vi "All IOs.vi"() -> ()   [LabVIEW 2015]
uses:
  <vilib>/rvi/Emulation/niFpgaGetClockAttributes.vi
  <vilib>/rvi/Emulation/niFpgaSctlEmulationGetInTimedLoop.vi
  <vilib>/rvi/Emulation/niFpgaEmulationReportErrorSimple.vi
  <vilib>/rvi/eio/common/nirviEmuTemplateMethod_errors.vi
  <vilib>/rvi/Emulation/niFpgaCriticalErrorInLSC.vi
  <vilib>/rvi/Emulation/niFpgaProcessEmulError.vi
  <vilib>/eio/EIONode/EIONode.xnode
panel:
  out "Time of flight":T1
  in  "6DOF robot arm controls":T2={"Axis  1 (base)"=1250, "Axis 2"=1600, "Axis 3"=1000, "Axis 4"=1900, "Axis 5"=1300, "Axis 6 (claw)"=1800} {"Axis 6 (claw)" min=500 max=2000; "Axis 5" min=500 max=2000; "Axis 4" min=500 max=2000; "Axis 3" min=500 max=2000; "Axis 2" min=500 max=2000; "Axis  1 (base)" min=500 max=2000}
  out "Lipo Battery Voltage":i16
  out "PIR 2":bool
  in  "FL":bool
  in  "BL":bool
  in  "FR":bool
  in  "BR":bool
  in  "On-board LED Brightness":T3 {"LED3 Brightness" max=100; "LED2 Brightness" max=100; "LED1 Brightness" max=100; "LED0 Brightness" max=100}
  out "Accelerometer":T4
  out "Button0":bool
  out "PIR":bool
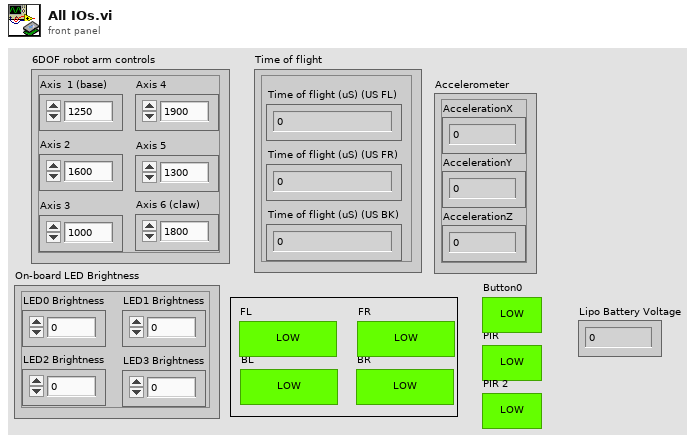
[diagram p1: front panel]
types:
  T1 = cluster{"Time of flight (uS) (US FL)":u32, "Time of flight (uS) (US FR)":u32, "Time of flight (uS) (US BK)":u32}
  T2 = cluster{"Axis  1 (base)":i16, "Axis 2":i16, "Axis 3":i16, "Axis 4":i16, "Axis 5":i16, "Axis 6 (claw)":i16}
  T3 = cluster{"LED0 Brightness":u8, "LED1 Brightness":u8, "LED2 Brightness":u8, "LED3 Brightness":u8}
  T4 = cluster{"AccelerationX":i16, "AccelerationY":i16, "AccelerationZ":i16}
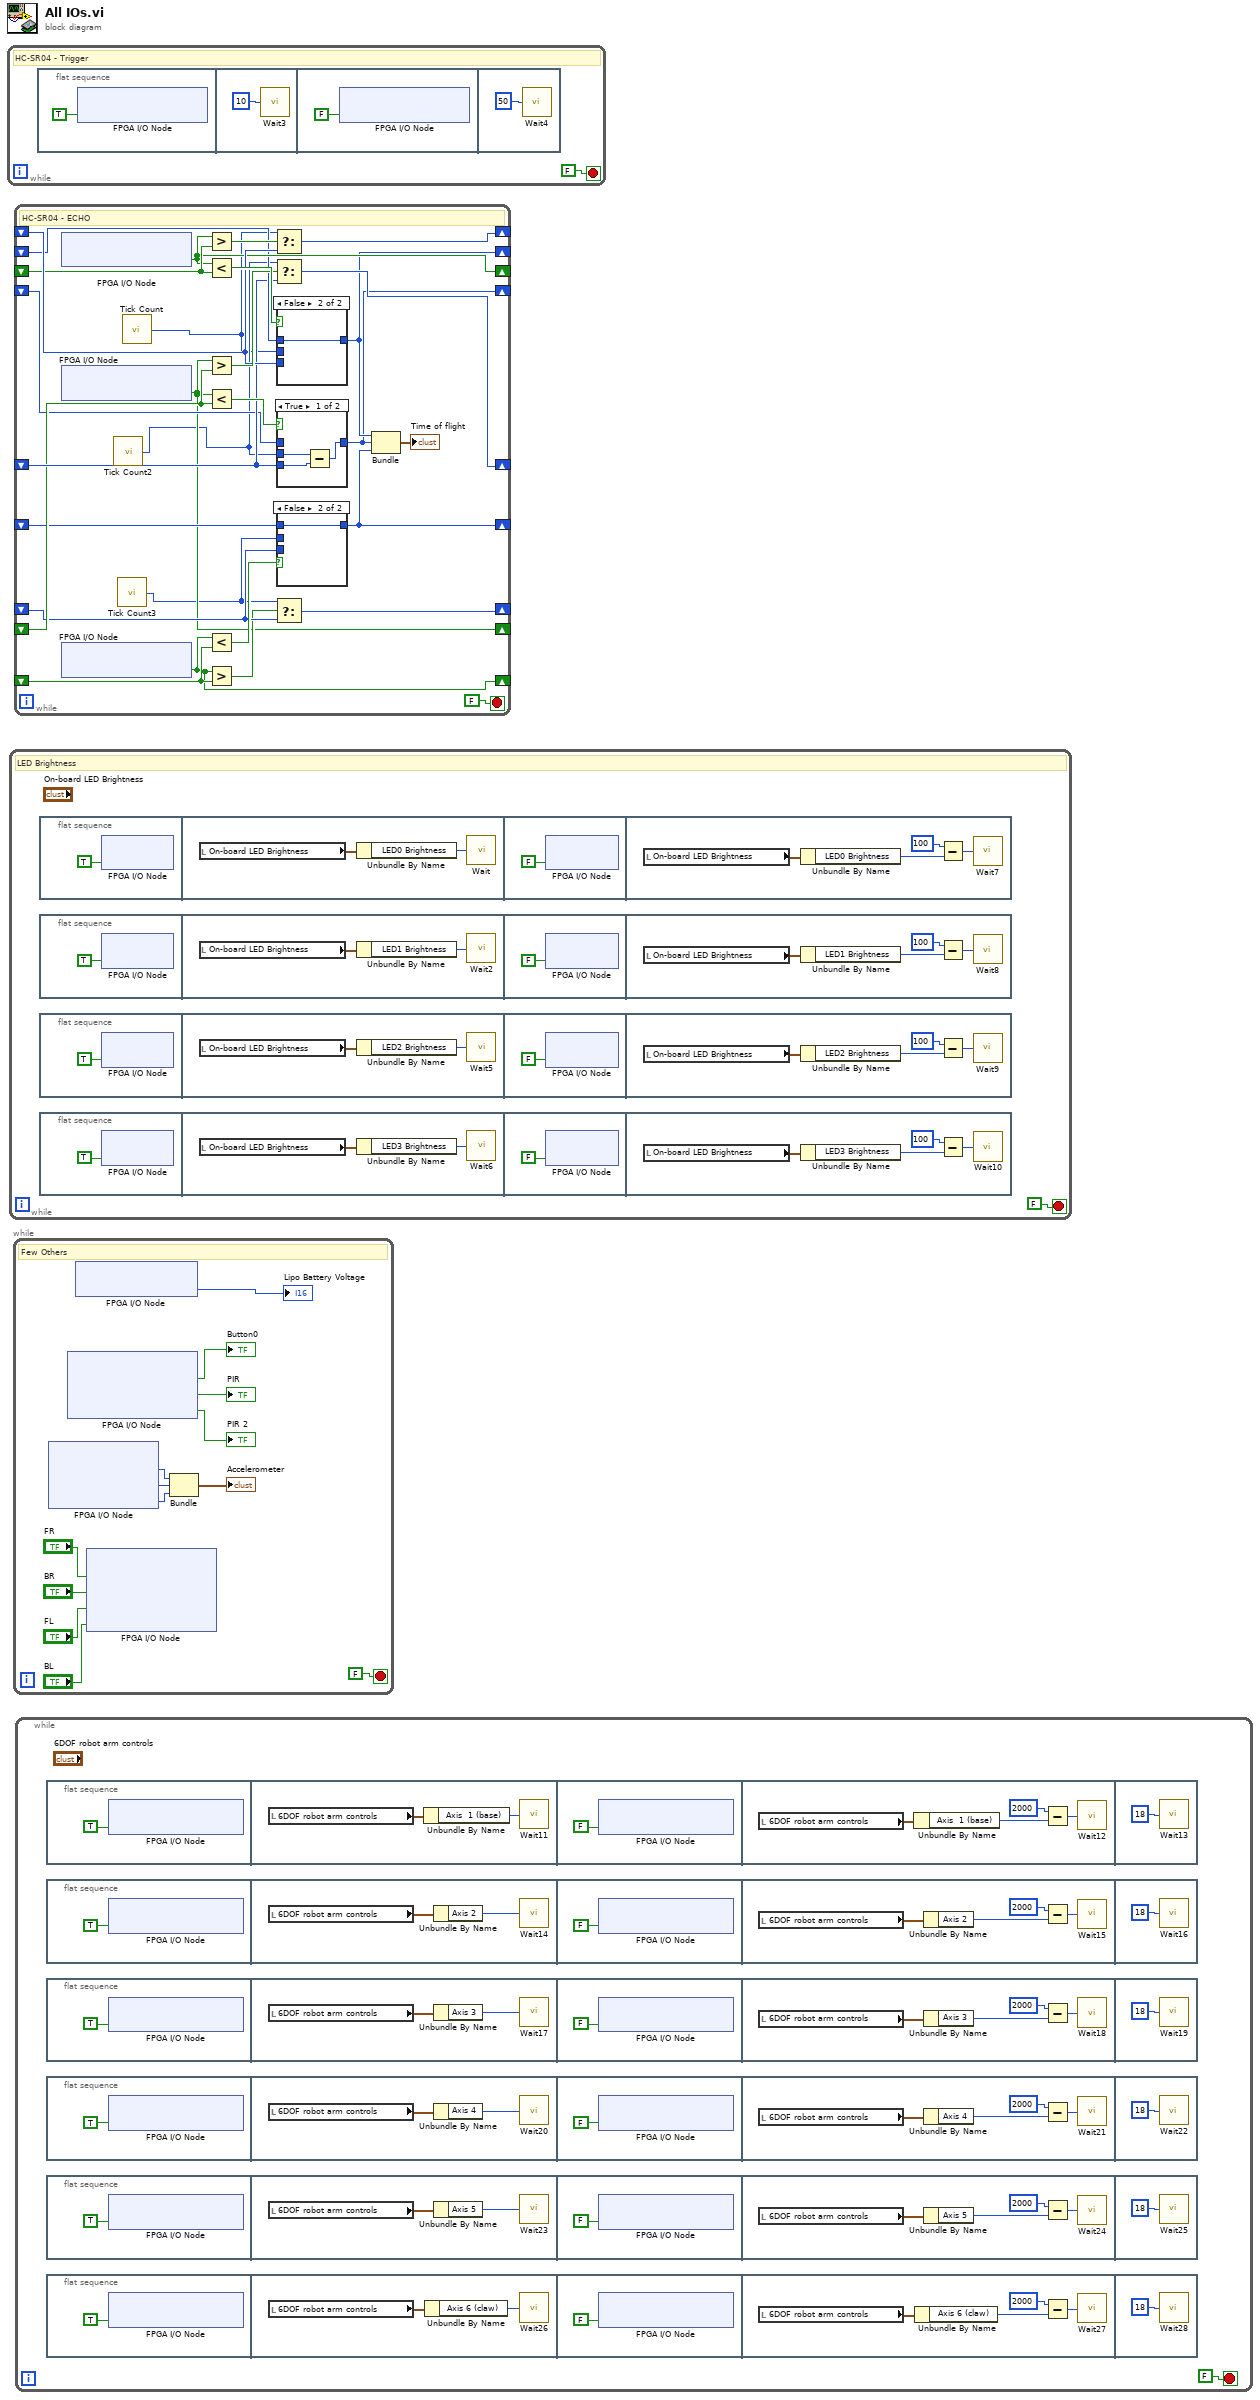
[diagram p0: block diagram]
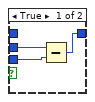
[diagram p2: hidden frame]
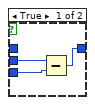
[diagram p3: hidden frame]
diagram:
  n1 = while {
    stop <- FALSE stop-if-true
    # "HC-SR04 - Trigger"
    n2 = flat-sequence {
      frame #0 {
        n3 = xnode "FPGA I/O Node"("ConnectorC/DIO0"=TRUE ("ConnectorC/DIO6")) -> ()  [unwired: 1 in, 1 out]
      }
      frame #1 {
        n4 = call "Wait3"("Count(uSec)"=u32 10) -> ()  [unwired: 1 out]
      }
      frame #2 {
        n5 = xnode "FPGA I/O Node"("ConnectorC/DIO0"=FALSE ("ConnectorC/DIO6")) -> ()  [unwired: 1 in, 1 out]
      }
      frame #3 {
        n6 = call "Wait4"("Count(mSec)"=i16 50) -> ()  [unwired: 1 out]
      }
    }
  }
  n7 = while {
    stop <- FALSE stop-if-true
    # "LED Brightness"
    n8 = flat-sequence {
      frame #0 {
        n9 = xnode "FPGA I/O Node"("LED0"=TRUE) -> ()  [unwired: 1 in, 1 out]
      }
      frame #1 {
        n10 = local read "On-board LED Brightness"() -> (w33:T3)
        n11 = Unbundle By Name(w33) -> ("LED0 Brightness"=w32:u8)
        n12 = call "Wait"("Count(uSec)"=w32) -> ()  [unwired: 1 out]
      }
      frame #2 {
        n13 = xnode "FPGA I/O Node"("LED0"=FALSE) -> ()  [unwired: 1 in, 1 out]
      }
      frame #3 {
        n14 = local read "On-board LED Brightness"() -> (w38:T3)
        n15 = Unbundle By Name(w38) -> ("LED0 Brightness"=w35:u8)
        n16 = Subtract(x=i16 100, y=w35) -> (x-y=w37:i16)
        n17 = call "Wait7"("Count(uSec)"=w37) -> ()  [unwired: 1 out]
      }
    }
    n18 = flat-sequence {
      frame #0 {
        n19 = xnode "FPGA I/O Node"("LED1"=TRUE) -> ()  [unwired: 1 in, 1 out]
      }
      frame #1 {
        n20 = local read "On-board LED Brightness"() -> (w24:T3)
        n21 = Unbundle By Name(w24) -> ("LED1 Brightness"=w25:u8)
        n22 = call "Wait2"("Count(uSec)"=w25) -> ()  [unwired: 1 out]
      }
      frame #2 {
        n23 = xnode "FPGA I/O Node"("LED1"=FALSE) -> ()  [unwired: 1 in, 1 out]
      }
      frame #3 {
        n24 = local read "On-board LED Brightness"() -> (w30:T3)
        n25 = Unbundle By Name(w30) -> ("LED1 Brightness"=w29:u8)
        n26 = Subtract(x=i16 100, y=w29) -> (x-y=w28:i16)
        n27 = call "Wait8"("Count(uSec)"=w28) -> ()  [unwired: 1 out]
      }
    }
    n28 = flat-sequence {
      frame #0 {
        n29 = xnode "FPGA I/O Node"("LED2"=TRUE) -> ()  [unwired: 1 in, 1 out]
      }
      frame #1 {
        n30 = local read "On-board LED Brightness"() -> (w17:T3)
        n31 = Unbundle By Name(w17) -> ("LED2 Brightness"=w16:u8)
        n32 = call "Wait5"("Count(uSec)"=w16) -> ()  [unwired: 1 out]
      }
      frame #2 {
        n33 = xnode "FPGA I/O Node"("LED2"=FALSE) -> ()  [unwired: 1 in, 1 out]
      }
      frame #3 {
        n34 = local read "On-board LED Brightness"() -> (w22:T3)
        n35 = Unbundle By Name(w22) -> ("LED2 Brightness"=w19:u8)
        n36 = Subtract(x=i16 100, y=w19) -> (x-y=w21:i16)
        n37 = call "Wait9"("Count(uSec)"=w21) -> ()  [unwired: 1 out]
      }
    }
    n38 = flat-sequence {
      frame #0 {
        n39 = xnode "FPGA I/O Node"("LED3"=TRUE) -> ()  [unwired: 1 in, 1 out]
      }
      frame #1 {
        n40 = local read "On-board LED Brightness"() -> (w8:T3)
        n41 = Unbundle By Name(w8) -> ("LED3 Brightness"=w9:u8)
        n42 = call "Wait6"("Count(uSec)"=w9) -> ()  [unwired: 1 out]
      }
      frame #2 {
        n43 = xnode "FPGA I/O Node"("LED3"=FALSE) -> ()  [unwired: 1 in, 1 out]
      }
      frame #3 {
        n44 = local read "On-board LED Brightness"() -> (w14:T3)
        n45 = Unbundle By Name(w14) -> ("LED3 Brightness"=w11:u8)
        n46 = Subtract(x=i16 100, y=w11) -> (x-y=w13:i16)
        n47 = call "Wait10"("Count(uSec)"=w13) -> ()  [unwired: 1 out]
      }
    }
  }
  n48 = while {
    stop <- FALSE stop-if-true
    # "Few Others"
    n49 = xnode "FPGA I/O Node"() -> ("AccelerationX"=w51:i16, "AccelerationY"=w50:i16, "AccelerationZ"=w49:i16)  [unwired: 3 in, 3 out]
    n50 = xnode "FPGA I/O Node"() -> ("Button0"=→"Button0":bool, "ConnectorB/DIO4"=→"PIR":bool, "ConnectorB/DIO5"=→"PIR 2":bool)  [unwired: 3 in, 3 out]
    n51 = xnode "FPGA I/O Node"() -> ("ConnectorC/AI0"=→"Lipo Battery Voltage":i16)  [unwired: 1 in, 1 out]
    n52 = xnode "FPGA I/O Node"("ConnectorB/DIO0"="FR", "ConnectorB/DIO1"="BR", "ConnectorB/DIO2"="FL", "ConnectorB/DIO3"="BL") -> ()  [unwired: 4 in, 4 out]
    n53 = Bundle("AccelerationX"=w51, "AccelerationY"=w50, "AccelerationZ"=w49) -> (→"Accelerometer":T4)  [unwired: 1 in]
  }
  n54 = while {
    shift-right: [w74] -> _
    shift-left: _ -> [w75]
    shift-right: [w72] -> _
    shift-left: _ -> [w73]
    shift-right: [w58] -> _
    shift-left: _ -> [w71]
    shift-right: [w67] -> _
    shift-left: _ -> [w70]
    shift-right: [w61] -> _
    shift-left: _ -> [w69]
    shift-right: [w57] -> _
    shift-left: _ -> [w68]
    shift-right: [w56] -> _
    shift-left: _ -> [w66]
    shift-right: [w64] -> _
    shift-left: _ -> [w65]
    shift-right: [w60] -> _
    shift-left: _ -> [w63]
    stop <- FALSE stop-if-true
    # "HC-SR04 - ECHO"
    n55 = xnode "FPGA I/O Node"() -> ("ConnectorC/DIO1"=w72:bool)  [unwired: 1 in, 1 out]
    n56 = xnode "FPGA I/O Node"() -> ("ConnectorC/DIO2"=w61:bool)  [unwired: 1 in, 1 out]
    n57 = xnode "FPGA I/O Node"() -> ("ConnectorC/DIO3"=w60:bool)  [unwired: 1 in, 1 out]
    n58 = call "Tick Count2"() -> ("Tick Count(uSec)"=w53:u32)
    n59 = call "Tick Count3"() -> ("Tick Count(uSec)"=w54:u32)
    n60 = call "Tick Count"() -> ("Tick Count(uSec)"=w52:u32)
    n61 = Greater?(x=w72, y=w73) -> (0:w79:bool)
    n62 = Less?(x=w72, y=w73) -> (x < y?=w78:bool)
    n63 = Greater?(x=w61, y=w69) -> (0:w77:bool)
    n64 = Less?(x=w61, y=w69) -> (x < y?=w76:bool)
    n65 = Less?(x=w60, y=w63) -> (x < y?=w80:bool)
    n66 = Greater?(x=w60, y=w63) -> (0:w62:bool)
    n67 = Select(t=w52, s=w79, f=w75) -> (s? t:f=w74:u32)
    n68 = Select(t=w53, s=w77, f=w70) -> (s? t:f=w67:u32)
    n69 = Select(t=w54, s=w62, f=w65) -> (s? t:f=w64:u32)
    n70 = case shown="False" w78 {
      tunnel: w71 -> [_ w88]
      tunnel: w52 -> [w85 _]
      tunnel: w75 -> [w86 _]
      tunnel: [w87 w88] -> w58
      frame True {
        n71 = Subtract(x=w85, y=w86) -> (x-y=w87:u32)
      }
      frame False {
      }
    }
    n72 = case shown="True" w76 {
      tunnel: w68 -> [_ w92]
      tunnel: w53 -> [w89 _]
      tunnel: w70 -> [w90 _]
      tunnel: [w91 w92] -> w57
      frame True {
        n73 = Subtract(x=w89, y=w90) -> (x-y=w91:u32)
      }
      frame False {
      }
    }
    n74 = case shown="False" w80 {
      tunnel: w66 -> [_ w84]
      tunnel: w54 -> [w81 _]
      tunnel: w65 -> [w82 _]
      tunnel: [w83 w84] -> w56
      frame True {
        n75 = Subtract(x=w81, y=w82) -> (x-y=w83:u32)
      }
      frame False {
      }
    }
    n76 = Bundle(w58, w57, w56) -> (→"Time of flight":cluster{u32, u32, u32})  [unwired: 1 in]
  }
  n77 = while {
    stop <- FALSE stop-if-true
    n78 = flat-sequence {
      frame #0 {
        n79 = xnode "FPGA I/O Node"("ConnectorB/DIO10"=TRUE) -> ()  [unwired: 1 in, 1 out]
      }
      frame #1 {
        n80 = local read "6DOF robot arm controls"() -> (w132:T2)
        n81 = Unbundle By Name(w132) -> ("Axis  1 (base)"=w131:i16)
        n82 = call "Wait11"("Count(uSec)"=w131) -> ()  [unwired: 1 out]
      }
      frame #2 {
        n83 = xnode "FPGA I/O Node"("ConnectorB/DIO10"=FALSE) -> ()  [unwired: 1 in, 1 out]
      }
      frame #3 {
        n84 = local read "6DOF robot arm controls"() -> (w135:T2)
        n85 = Unbundle By Name(w135) -> ("Axis  1 (base)"=w134:i16)
        n86 = Subtract(x=i16 2000, y=w134) -> (x-y=w136:i16)
        n87 = call "Wait12"("Count(uSec)"=w136) -> ()  [unwired: 1 out]
      }
      frame #4 {
        n88 = call "Wait13"("Count(mSec)"=u32 18) -> ()  [unwired: 1 out]
      }
    }
    n89 = flat-sequence {
      frame #0 {
        n90 = xnode "FPGA I/O Node"("ConnectorB/DIO11"=TRUE) -> ()  [unwired: 1 in, 1 out]
      }
      frame #1 {
        n91 = local read "6DOF robot arm controls"() -> (w141:T2)
        n92 = Unbundle By Name(w141) -> ("Axis 2"=w140:i16)
        n93 = call "Wait14"("Count(uSec)"=w140) -> ()  [unwired: 1 out]
      }
      frame #2 {
        n94 = xnode "FPGA I/O Node"("ConnectorB/DIO11"=FALSE) -> ()  [unwired: 1 in, 1 out]
      }
      frame #3 {
        n95 = local read "6DOF robot arm controls"() -> (w144:T2)
        n96 = Unbundle By Name(w144) -> ("Axis 2"=w143:i16)
        n97 = Subtract(x=i16 2000, y=w143) -> (x-y=w145:i16)
        n98 = call "Wait15"("Count(uSec)"=w145) -> ()  [unwired: 1 out]
      }
      frame #4 {
        n99 = call "Wait16"("Count(mSec)"=u32 18) -> ()  [unwired: 1 out]
      }
    }
    n100 = flat-sequence {
      frame #0 {
        n101 = xnode "FPGA I/O Node"("ConnectorB/DIO12"=TRUE) -> ()  [unwired: 1 in, 1 out]
      }
      frame #1 {
        n102 = local read "6DOF robot arm controls"() -> (w123:T2)
        n103 = Unbundle By Name(w123) -> ("Axis 3"=w122:i16)
        n104 = call "Wait17"("Count(uSec)"=w122) -> ()  [unwired: 1 out]
      }
      frame #2 {
        n105 = xnode "FPGA I/O Node"("ConnectorB/DIO12"=FALSE) -> ()  [unwired: 1 in, 1 out]
      }
      frame #3 {
        n106 = local read "6DOF robot arm controls"() -> (w126:T2)
        n107 = Unbundle By Name(w126) -> ("Axis 3"=w125:i16)
        n108 = Subtract(x=i16 2000, y=w125) -> (x-y=w127:i16)
        n109 = call "Wait18"("Count(uSec)"=w127) -> ()  [unwired: 1 out]
      }
      frame #4 {
        n110 = call "Wait19"("Count(mSec)"=u32 18) -> ()  [unwired: 1 out]
      }
    }
    n111 = flat-sequence {
      frame #0 {
        n112 = xnode "FPGA I/O Node"("ConnectorB/DIO13"=TRUE) -> ()  [unwired: 1 in, 1 out]
      }
      frame #1 {
        n113 = local read "6DOF robot arm controls"() -> (w114:T2)
        n114 = Unbundle By Name(w114) -> ("Axis 4"=w113:i16)
        n115 = call "Wait20"("Count(uSec)"=w113) -> ()  [unwired: 1 out]
      }
      frame #2 {
        n116 = xnode "FPGA I/O Node"("ConnectorB/DIO13"=FALSE) -> ()  [unwired: 1 in, 1 out]
      }
      frame #3 {
        n117 = local read "6DOF robot arm controls"() -> (w117:T2)
        n118 = Unbundle By Name(w117) -> ("Axis 4"=w116:i16)
        n119 = Subtract(x=i16 2000, y=w116) -> (x-y=w118:i16)
        n120 = call "Wait21"("Count(uSec)"=w118) -> ()  [unwired: 1 out]
      }
      frame #4 {
        n121 = call "Wait22"("Count(mSec)"=u32 18) -> ()  [unwired: 1 out]
      }
    }
    n122 = flat-sequence {
      frame #0 {
        n123 = xnode "FPGA I/O Node"("ConnectorB/DIO14"=TRUE) -> ()  [unwired: 1 in, 1 out]
      }
      frame #1 {
        n124 = local read "6DOF robot arm controls"() -> (w105:T2)
        n125 = Unbundle By Name(w105) -> ("Axis 5"=w104:i16)
        n126 = call "Wait23"("Count(uSec)"=w104) -> ()  [unwired: 1 out]
      }
      frame #2 {
        n127 = xnode "FPGA I/O Node"("ConnectorB/DIO14"=FALSE) -> ()  [unwired: 1 in, 1 out]
      }
      frame #3 {
        n128 = local read "6DOF robot arm controls"() -> (w108:T2)
        n129 = Unbundle By Name(w108) -> ("Axis 5"=w107:i16)
        n130 = Subtract(x=i16 2000, y=w107) -> (x-y=w109:i16)
        n131 = call "Wait24"("Count(uSec)"=w109) -> ()  [unwired: 1 out]
      }
      frame #4 {
        n132 = call "Wait25"("Count(mSec)"=u32 18) -> ()  [unwired: 1 out]
      }
    }
    n133 = flat-sequence {
      frame #0 {
        n134 = xnode "FPGA I/O Node"("ConnectorB/DIO15"=TRUE) -> ()  [unwired: 1 in, 1 out]
      }
      frame #1 {
        n135 = local read "6DOF robot arm controls"() -> (w96:T2)
        n136 = Unbundle By Name(w96) -> ("Axis 6 (claw)"=w95:i16)
        n137 = call "Wait26"("Count(uSec)"=w95) -> ()  [unwired: 1 out]
      }
      frame #2 {
        n138 = xnode "FPGA I/O Node"("ConnectorB/DIO15"=FALSE) -> ()  [unwired: 1 in, 1 out]
      }
      frame #3 {
        n139 = local read "6DOF robot arm controls"() -> (w99:T2)
        n140 = Unbundle By Name(w99) -> ("Axis 6 (claw)"=w98:i16)
        n141 = Subtract(x=i16 2000, y=w98) -> (x-y=w100:i16)
        n142 = call "Wait27"("Count(uSec)"=w100) -> ()  [unwired: 1 out]
      }
      frame #4 {
        n143 = call "Wait28"("Count(mSec)"=u32 18) -> ()  [unwired: 1 out]
      }
    }
  }
